vi "Update Bind Method Constants.vi"(7 "RPC Method Parameters":T1, 8 "error in (no error)":errorcluster, 10 "RPC Method Name":string, 11 "VI in":refnum<vi>) -> (0 "error out":errorcluster, 3 "VI out":refnum<vi>)   [LabVIEW 2019, in "gRPC Template Creation Utility.lvlib"]
uses:
  gRPC Template Creation Utility.lvlib
  TypeDefs/RPC Method Parameters.ctl
  <vilib>/Utility/traverseref.llb/TRef TravTarget.ctl
  <vilib>/Utility/traverseref.llb/VI Scripting - Traverse.lvlib
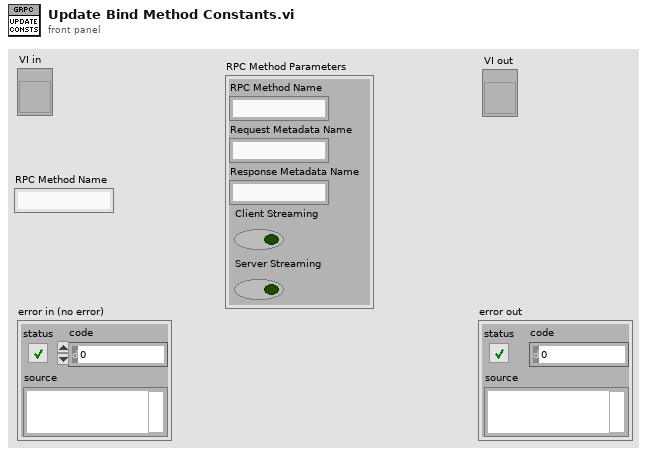
[diagram p1: front panel]
types:
  T1 = typedef "gRPC Template Creation Utility.lvlib/RPC Method Parameters.ctl" = cluster{"RPC Method Name":string, "Request Metadata Name":string, "Response Metadata Name":string, "Client Streaming":bool, "Server Streaming":bool}
  T2 = typedef "TRef TravTarget.ctl" = enum16{"FP", "BD", "Other"}
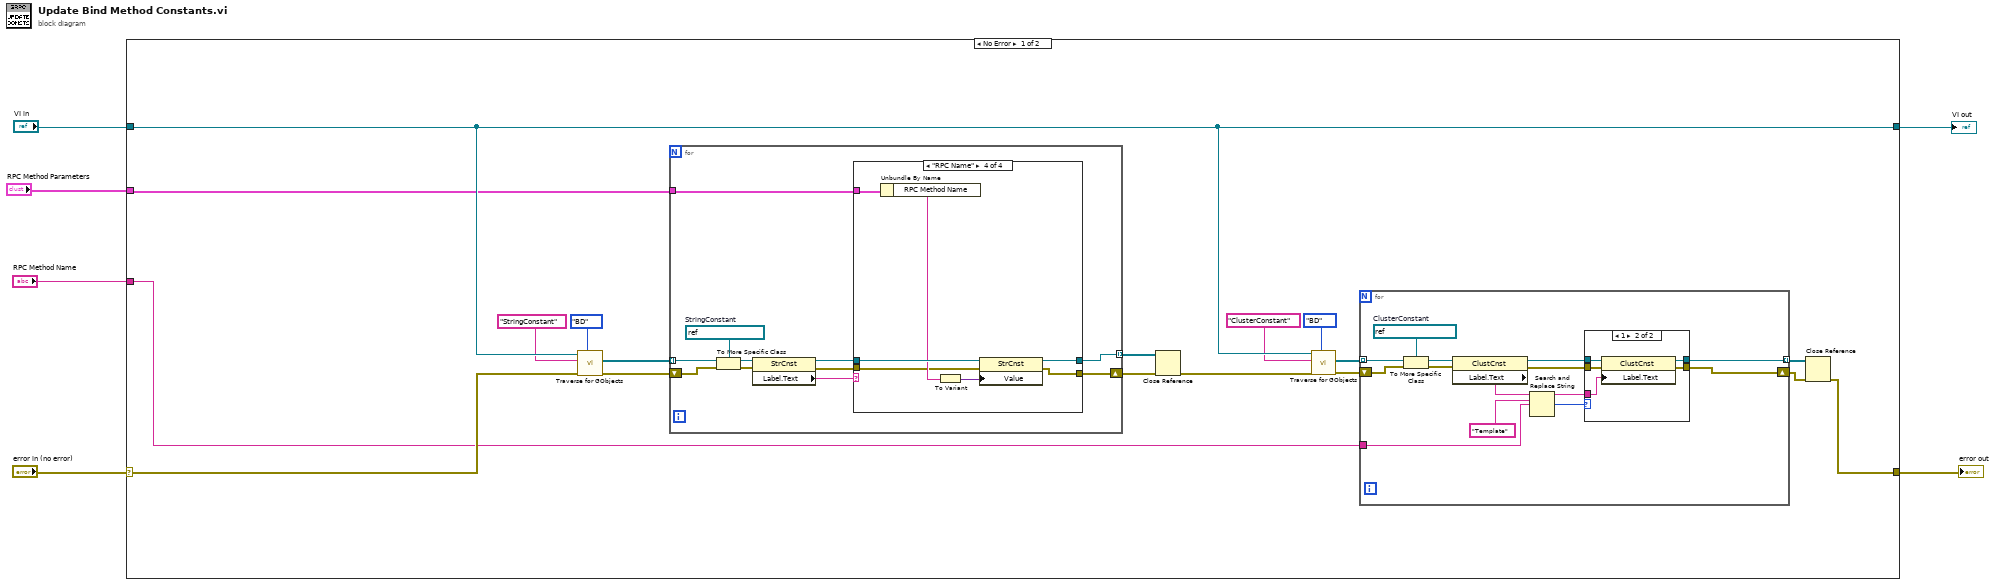
[diagram p0: block diagram]
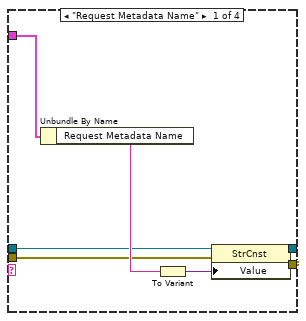
[diagram p3: hidden frame]
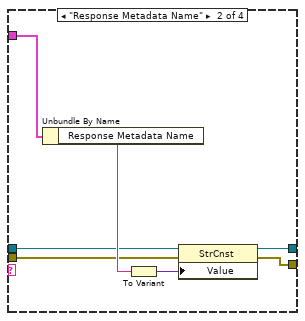
[diagram p4: hidden frame]
diagram:
  n1 = case shown="No Error" "error in (no error)" {
    selector: "error in (no error)" -> [w23 w81]
    tunnel: [w24 w81] -> w6
    tunnel: "VI in" -> [w22 w80]
    tunnel: "RPC Method Name" -> [w21 _]
    tunnel: [w22 w80] -> w2
    tunnel: "RPC Method Parameters" -> [w20 _]
    frame No Error {
      n2 = call <vilib>:"Traverse for GObjects.vi"("Traverse Target"=TRef_TravTarget."BD", "error in (no error)"=w23, "Class Name"="StringConstant", "VI Refnum"=w22) -> ("error out"=w17:errorcluster, "References"=w13:refnum<vi>[])  [unwired: 4 in, 2 out]
      n3 = for {
        tunnel: w13 -> [w55] mode=indexing
        shift-right: [w47] -> w14
        shift-left: w17 -> [w54]
        tunnel: w20 -> [w50]
        tunnel: [w46] -> w12 mode=indexing
        w56 = refnum<vi> refnum  # StringConstant
        n4 = To More Specific Class(target class=w56, reference=w55, error in=w54) -> (specific class reference=w53:refnum<vi>, error out=w52:errorcluster)
        n5 = property class="StrCnst"(reference=w53, error in=w52) -> (reference out=w49:refnum<vi>, error out=w48:errorcluster, "Label.Text"=w51:string)
        n6 = case shown="\"RPC Name\"" w51 {
          tunnel: w50 -> [w58 w68 _ w79]
          tunnel: w49 -> [w60 w66 w71 w78]
          tunnel: w48 -> [w61 w67 w72 w75]
          tunnel: [w59 w65 w72 w74] -> w47
          tunnel: [w57 w64 w71 w73] -> w46
          frame "Request Metadata Name" {
            n7 = Unbundle By Name(w58) -> ("Request Metadata Name"=w63:string)
            n8 = To Variant(anything=w63) -> (Variant=w62:variant)
            n9 = property class="StrCnst"(reference=w60, error in=w61, "Value"=w62) -> (reference out=w57:refnum<vi>, error out=w59:errorcluster)
          }
          frame "Response Metadata Name" {
            n10 = Unbundle By Name(w68) -> ("Response Metadata Name"=w70:string)
            n11 = To Variant(anything=w70) -> (Variant=w69:variant)
            n12 = property class="StrCnst"(reference=w66, error in=w67, "Value"=w69) -> (reference out=w64:refnum<vi>, error out=w65:errorcluster)
          }
          frame "None", Default {
          }
          frame "RPC Name" {
            n13 = Unbundle By Name(w79) -> ("RPC Method Name"=w77:string)
            n14 = To Variant(anything=w77) -> (Variant=w76:variant)
            n15 = property class="StrCnst"(reference=w78, error in=w75, "Value"=w76) -> (reference out=w73:refnum<vi>, error out=w74:errorcluster)
          }
        }
      }
      n16 = Close Reference(reference=w12, error in (no error)=w14) -> (error out=w11:errorcluster)
      n17 = call <vilib>:"Traverse for GObjects.vi"("Traverse Target"=TRef_TravTarget."BD", "error in (no error)"=w11, "Class Name"="ClusterConstant", "VI Refnum"=w22) -> ("error out"=w10:errorcluster, "References"=w9:refnum<vi>[])  [unwired: 4 in, 2 out]
      n18 = for {
        tunnel: w9 -> [w37] mode=indexing
        shift-right: [w26] -> w8
        shift-left: w10 -> [w36]
        tunnel: w21 -> [w31]
        tunnel: [w25] -> w7 mode=indexing
        w38 = refnum<vi> refnum  # ClusterConstant
        n19 = To More Specific Class(target class=w38, reference=w37, error in=w36) -> (specific class reference=w35:refnum<vi>, error out=w34:errorcluster)
        n20 = property class="ClustCnst"(reference=w35, error in=w34) -> (reference out=w30:refnum<vi>, error out=w29:errorcluster, "Label.Text"=w32:string)
        n21 = Search and Replace String(input string=w32, search string="Template", replace string=w31) -> (result string=w27:string, number of replacements=w28:i32)  [unwired: 5 in, 2 out]
        n22 = case shown="1" w28 {
          tunnel: w30 -> [w40 w45]
          tunnel: [w40 w44] -> w25
          tunnel: [w39 w43] -> w26
          tunnel: w29 -> [w39 w42]
          tunnel: w27 -> [_ w41]
          frame 0, Default {
          }
          frame 1 {
            n23 = property class="ClustCnst"(reference=w45, error in=w42, "Label.Text"=w41) -> (reference out=w44:refnum<vi>, error out=w43:errorcluster)
          }
        }
      }
      n24 = Close Reference(reference=w7, error in (no error)=w8) -> (error out=w24:errorcluster)
    }
    frame Error {
    }
  }
  "error out" <- w6
  "VI out" <- w2
